vi "FRCts20_Backend_Stats_GET_reform.vi"(6 "Special Device Usage":variant[][](array[variant]), 8 "Error In":errorcluster, 9 "SW usage - Live Events":variant[][](array[variant]), 10 "Global SW Info":variant[][](array[variant]), 11 "Requests Per Hour":variant[][](array[variant])) -> (0 "Error Out":errorcluster, 3 "data string":string)   [LabVIEW 2014, in "FRCts20_Backend_Engine.lvlib"]
uses:
  FRCts20_Backend_Engine.lvlib
  FRCts20_Backend_API/FRCts20_Backend_API_Stats.ctl
  ESP Engine/source/VI Source/TypeDefs/FRCts20_EspEngine_RequestPerHour_Line.ctl
  ESP Engine/source/VI Source/TypeDefs/FRCts20_EspEngine_SwUsage_Pie.ctl
  ESP Engine/source/VI Source/TypeDefs/FRCts20_EspEngine_AdvancedComponents_Bar.ctl
  <vilib>/addons/database/_DB Variant To Data/Database Variant To Data.xnode
  ESP Engine/source/VI Source/FRCts20_EspEngine.lvlib
  FRCts20_Backend_API/FRCts20_Backend_API.lvlib
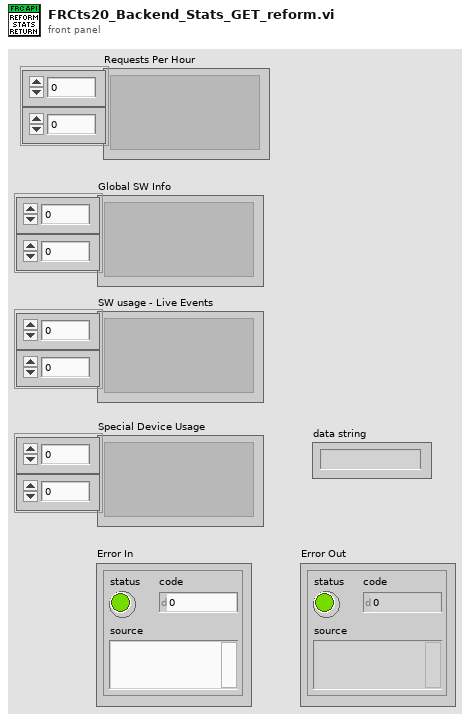
[diagram p1: front panel]
types:
  T1 = cluster{"eventName":string, "startYear":i32, "startHour":i32, "startDay":i32, "numRequests":i32, "requestHour":i32}[]
  T2 = cluster{"EventName":string, "SWType":string, "Number":dbl}[]
  T3 = typedef "FRCts20_EspEngine.lvlib/FRCts20_EspEngine_AdvancedComponents_Bar.ctl" = cluster{"CAN":i32, "Vision":i32, "Kinect":i32}
  T4 = typedef "FRCts20_Backend_API.lvlib/FRCts20_Backend_API_Stats.ctl" = cluster{"RequestsPerHour":T5, "SW Usage Pies":T6, "Advanced Components":T3, "APIReturn":string}
  T5 = typedef "FRCts20_EspEngine.lvlib/FRCts20_EspEngine_RequestPerHour_Line.ctl" = cluster{"StartDate":cluster{"Year":i32, "Month":i32, "Day":i32}, "Events":cluster{"Location":string, "Requests":i32[]}[]}
  T6 = typedef "FRCts20_EspEngine.lvlib/FRCts20_EspEngine_SwUsage_Pie.ctl" = cluster{"Live Event Location":string, "LabVIEW":dbl, "C++":dbl, "Java":dbl, "Other":dbl, "TotalTeams":i32, "TeamsReporting":i32}[]
  T7 = cluster{"Live Event Location":string, "LabVIEW":dbl, "C++":dbl, "Java":dbl, "Other":dbl, "TotalTeams":i32, "TeamsReporting":i32}
  T8 = cluster{"Live Event Location":string, "LabVIEW":dbl, "C++":dbl, "Java":dbl, "Other":dbl, "TotalTeams":i32, "TeamsReporting":i32}[]
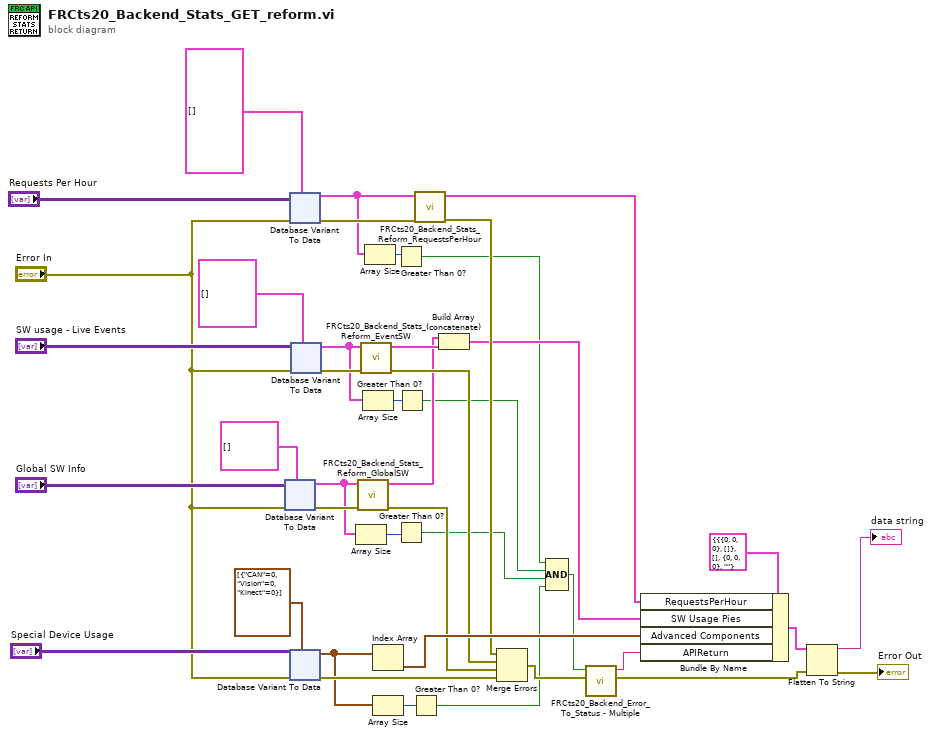
[diagram p0: block diagram]
diagram:
  n1 = xnode "Database Variant To Data"("database variant"="Global SW Info", "error in (no error)"="Error In", "type"=cluster{"SWType":string, "Number":dbl}[] []) -> ("data"=w18:cluster{"SWType":string, "Number":dbl}[], "error out"=w23:errorcluster)
  n2 = xnode "Database Variant To Data"("database variant"="Requests Per Hour", "error in (no error)"="Error In", "type"=T1 []) -> ("data"=w13:T1, "error out"=w16:errorcluster)
  n3 = xnode "Database Variant To Data"("database variant"="Special Device Usage", "error in (no error)"="Error In", "type"=T3[] [{"CAN"=0, "Vision"=0, "Kinect"=0}]) -> ("data"=w27:T3[], "error out"=w29:errorcluster)
  n4 = xnode "Database Variant To Data"("database variant"="SW usage - Live Events", "error in (no error)"="Error In", "type"=T2 []) -> ("data"=w19:T2, "error out"=w22:errorcluster)
  n5 = Array Size(array=w18) -> (size(s)=w6:i32)
  n6 = call "FRCts20_Backend_Stats_Reform_GlobalSW.vi"("Error In"=w23, "data"=w18) -> ("Error Out"=w21:errorcluster, "Software Usage Pie"=w11:T7)  [unwired: 8 in]
  n7 = call "FRCts20_Backend_Stats_Reform_EventSW.vi"("Error In"=w22, "data"=w19) -> ("Error Out"=w20:errorcluster, "Array"=w12:T8)  [unwired: 8 in]
  n8 = Array Size(array=w19) -> (size(s)=w4:i32)
  n9 = Array Size(array=w13) -> (size(s)=w2:i32)
  n10 = Index Array(array=w27) -> (element=w31:T3)  [unwired: 1 in]
  n11 = Array Size(array=w27) -> (size(s)=w9:i32)
  n12 = Greater Than 0?(x=w2) -> (x > 0?=w1:bool)
  n13 = Greater Than 0?(x=w6) -> (x > 0?=w5:bool)
  n14 = Greater Than 0?(x=w4) -> (x > 0?=w3:bool)
  n15 = Greater Than 0?(x=w9) -> (x > 0?=w8:bool)
  n16 = call "FRCts20_Backend_Stats_Reform_RequestsPerHour.vi"("error in (no error)"=w16, "Array"=w13) -> ("Error Out"=w14:errorcluster, "RequestsPerHour"=w15:T5)  [unwired: 8 in]
  n17 = Build Array (concatenate)(w11, w12) -> (w10:T8)
  n18 = Merge Errors(w14, w20, w21, w29) -> (w28:errorcluster)
  n19 = Compound Arithmetic op=AND(w1, w3, w5, w8) -> (w7:bool)
  n20 = call "FRCts20_Backend_Error_To_Status - Multiple.vi"("error in (no error)"=w28, "rows affected?"=w7) -> ("error out"=w34:errorcluster, "String"=w35:string)  [unwired: 8 in]
  n21 = Bundle By Name(cluster=T4 {"RequestsPerHour"={"StartDate"={"Year"=0, "Month"=0, "Day"=0}, "Events"=[]}, "SW Usage Pies"=[], "Advanced Components"={"CAN"=0, "Vision"=0, "Kinect"=0}, "APIReturn"=""} ("Statistics"), "RequestsPerHour"=w15, "SW Usage Pies"=w10, "Advanced Components"=w31, "APIReturn"=w35) -> (w33:T4)
  n22 = Flatten To String(anything=w33, error in (no error)=w34) -> (data string=→"data string":string, error out=→"Error Out":errorcluster)  [unwired: 2 in, 1 out]
